vi "itc Hg box controller.vi"(6 "Log File Path":path, 7 "itc box action":T2=enum."read sweep table", 8 "error in":errorcluster, 9 "Sweep Table In":dbl[][](array[numeric])=[[650.0, 1334.0, 30.0], [300.0, 1334.0, 0.0], [0.0, 0.0, 0.0], [0.0, 0.0, 0.0], [0.0, 0.0, 0.0], [0.0, 0.0, 0.0], [0.0, 0.0, 0.0], [0.0, 0.0, 0.0], [0.0, 0.0, 0.0], [0.0, 0.0, 0.0], [0.0, 0.0, 0.0], [300.0, 0.0, 0.0], [0.0, 0.0, 0.0], [0.0, 0.0, 0.0], [0.0, 0.0, 0.0], [300.0, 0.0, 0.0]], 10 "input":dbl=300.0, 11 "VISA resource name":refnum<visa-resource-name>="GPIB0::23::INSTR") -> (0 "error out":errorcluster, 1 "Sweep Table":dbl[][](array[numeric])=[[650.0, 1334.0, 30.0], [300.0, 1334.0, 0.0], [0.0, 0.0, 0.0], [0.0, 0.0, 0.0], [0.0, 0.0, 0.0], [0.0, 0.0, 0.0], [0.0, 0.0, 0.0], [0.0, 0.0, 0.0], [0.0, 0.0, 0.0], [0.0, 0.0, 0.0], [0.0, 0.0, 0.0], [300.0, 0.0, 0.0], [0.0, 0.0, 0.0], [0.0, 0.0, 0.0], [0.0, 0.0, 0.0], [300.0, 0.0, 0.0]], 2 "itc box state OUT":T1={"ITC503 Address"="GPIB0::15::INSTR", "ITC temperature"=0.0, "ITC set temperature"=300.0, "heater"=300.0, "gas flow"=1.6, "P"=0.0, "D"=10.0, "I"=0.1, "ITC state"="X0A1C2S01H1L0\r", "nonzero temperature"=0.0, "Magn Field (T)"=0.0})   [LabVIEW 2015]
uses:
  itc 503 box - control.ctl
  itc 503 box state.ctl
  Q - not nan -- real.vi
panel:
  out "F-format string":string
  out "enabled state":enum16{"disabled", "enabled"}(ring)
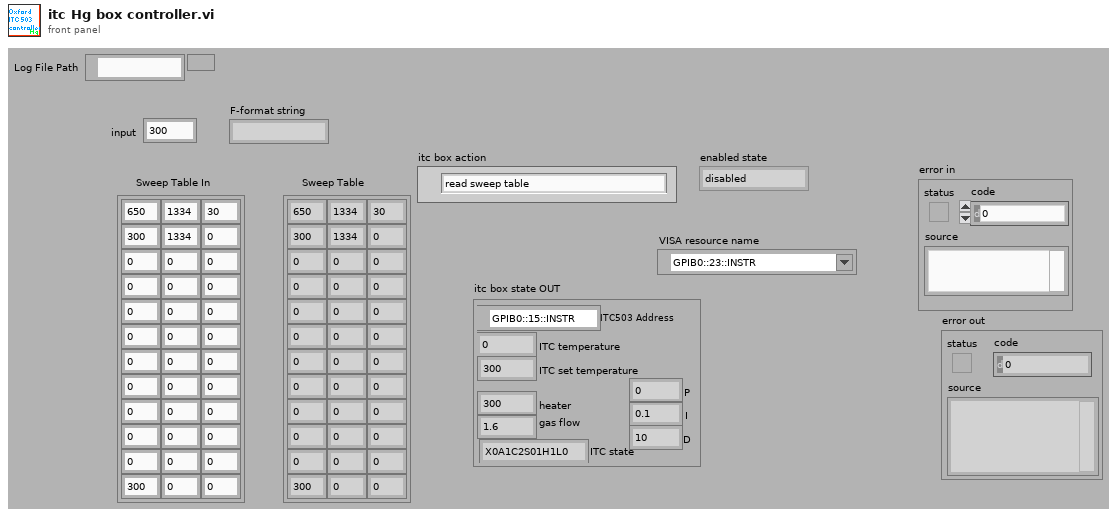
[diagram p1: front panel]
types:
  T1 = typedef "itc 503 box state.ctl" = cluster{"ITC503 Address":refnum<visa-resource-name>, "ITC temperature":dbl, "ITC set temperature":dbl, "heater":dbl, "gas flow":dbl, "P":dbl, "D":dbl, "I":dbl, "ITC state":string, "nonzero temperature":dbl, "Magn Field (T)":dbl}
  T2 = typedef "itc 503 box - control.ctl" = enum16{"heater manual and zero", "heater auto", "upload D", "upload I", "upload P", "shut off", "init", "read sweep table", "disable", "enable", "read state", "set gas to", "stop sweep", "start sweep", "test", "set temperature to", "write sweep table", "-void", "set heater to"}
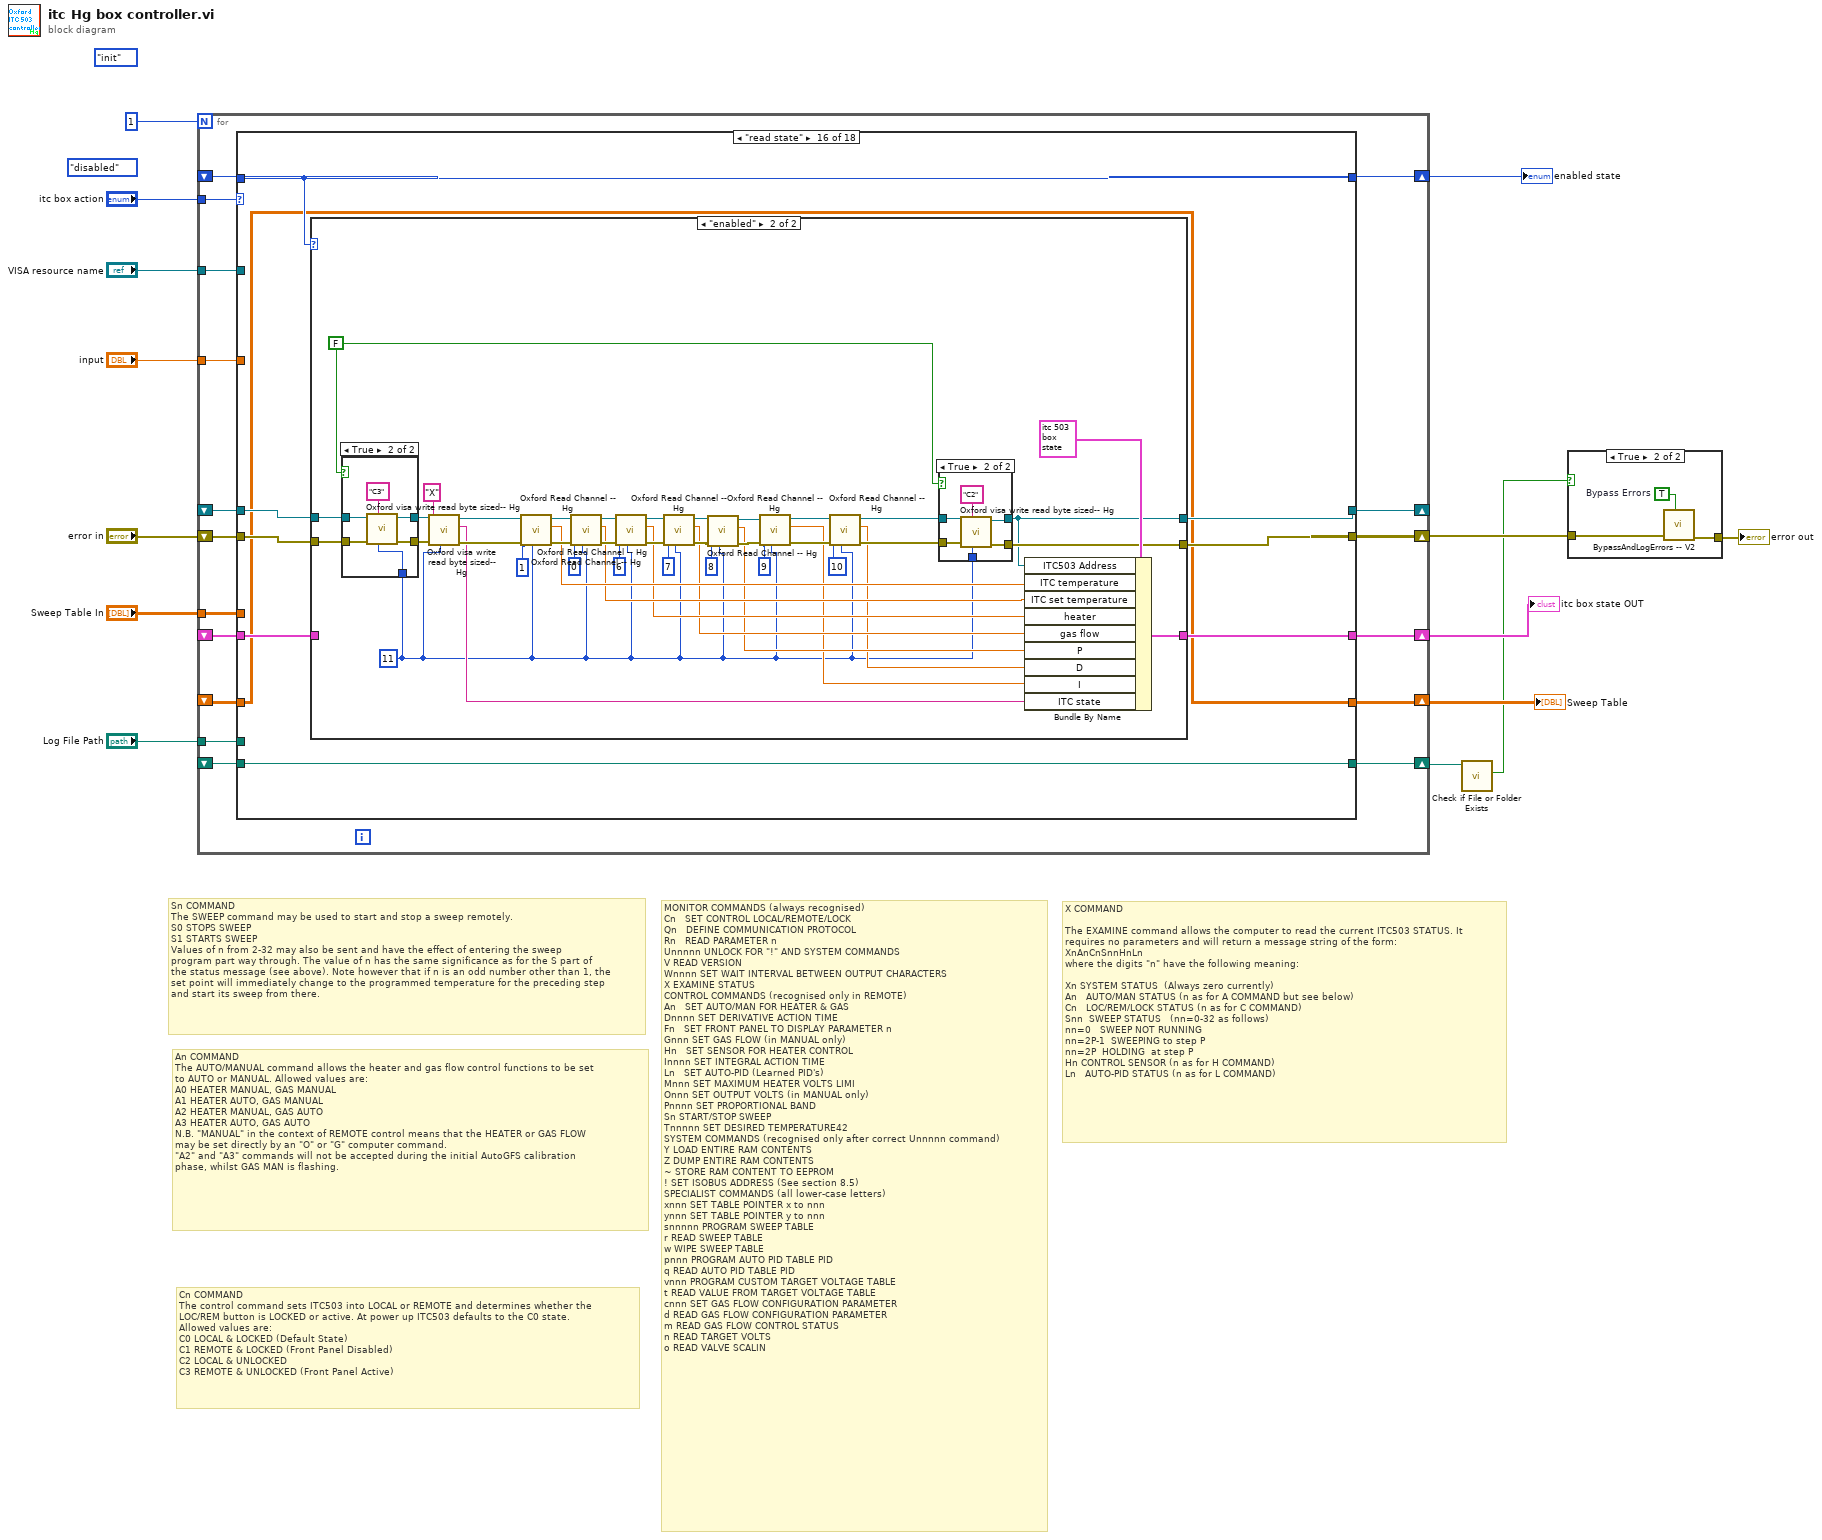
[diagram p0: block diagram]
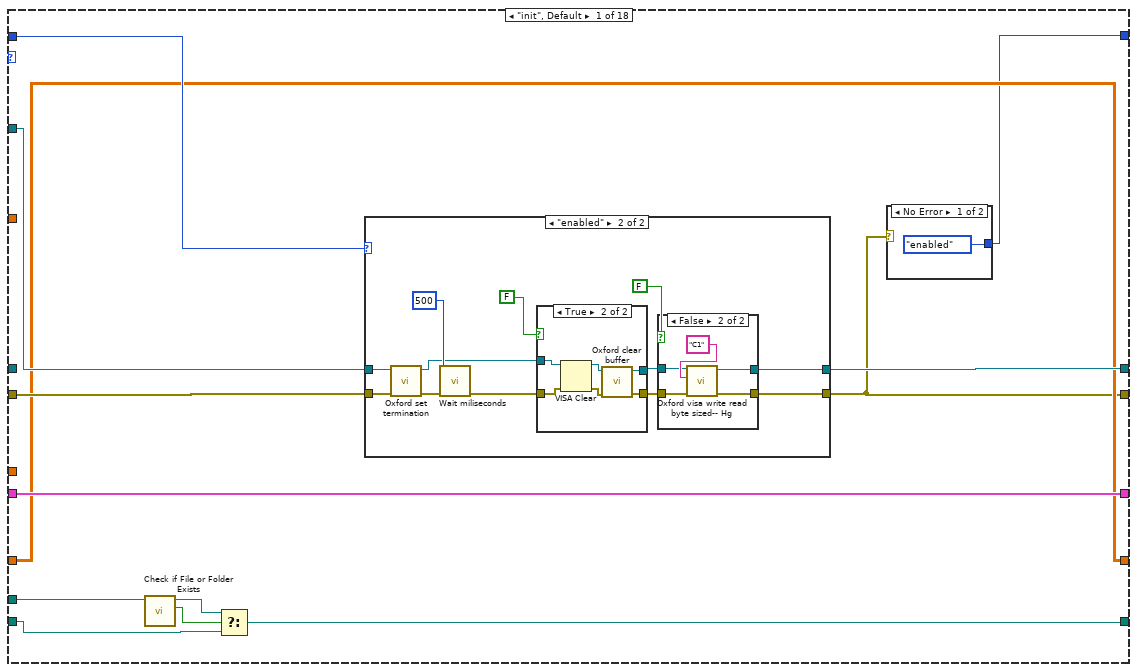
[diagram p3: hidden frame]
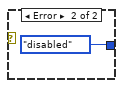
[diagram p4: hidden frame]
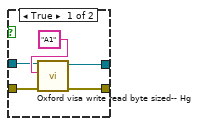
[diagram p7: hidden frame]
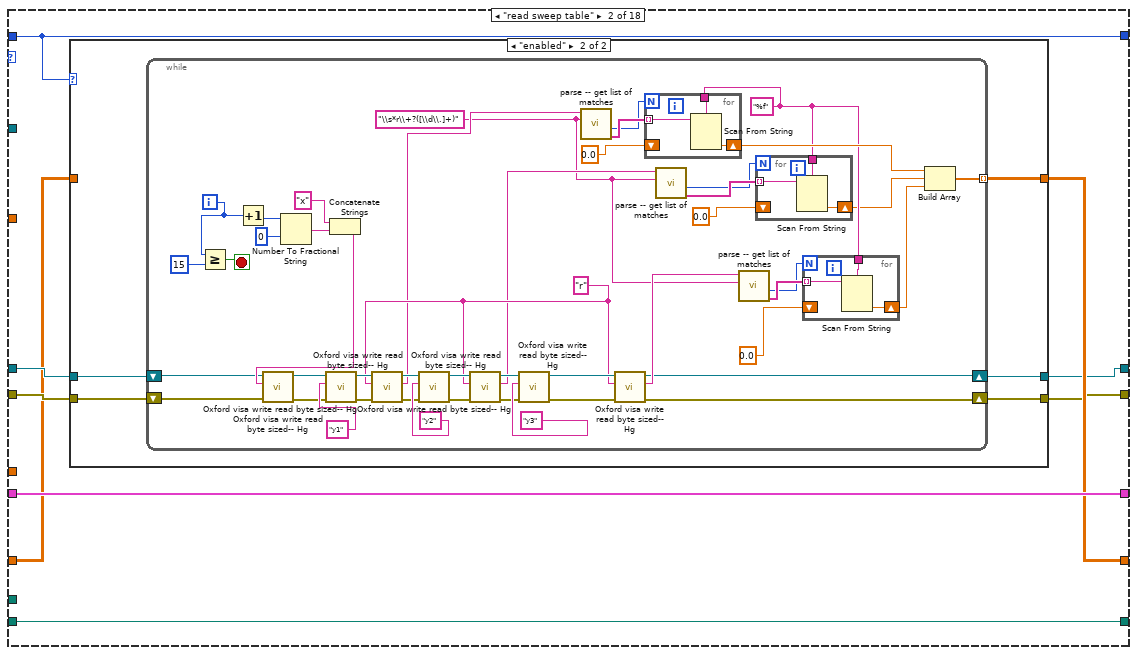
[diagram p8: hidden frame]
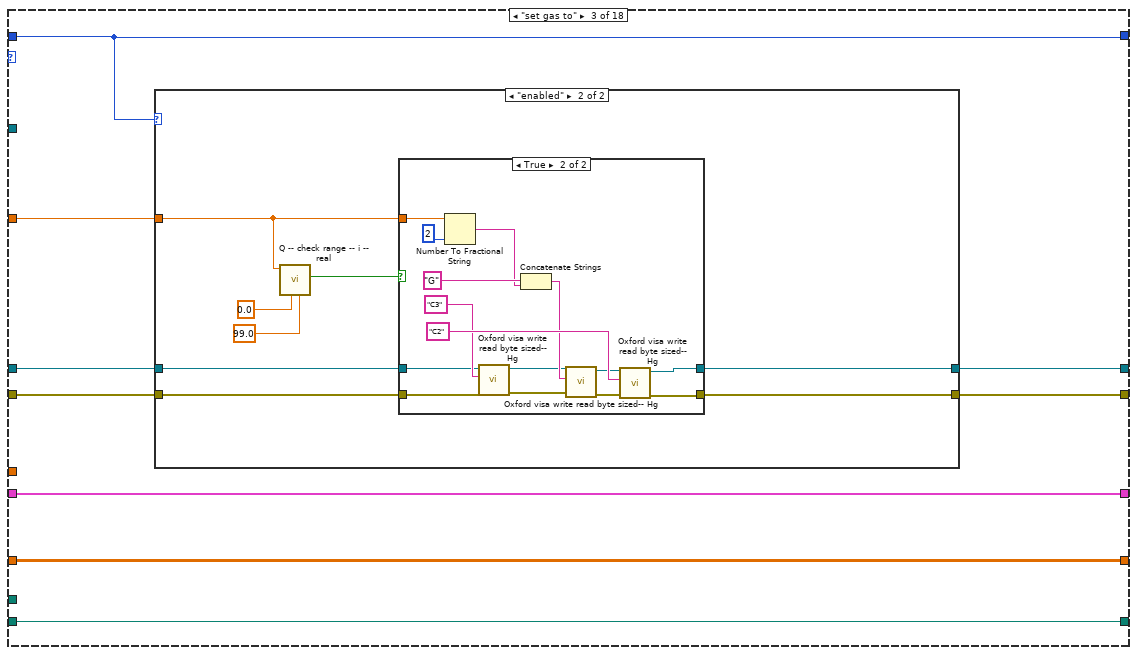
[diagram p10: hidden frame]
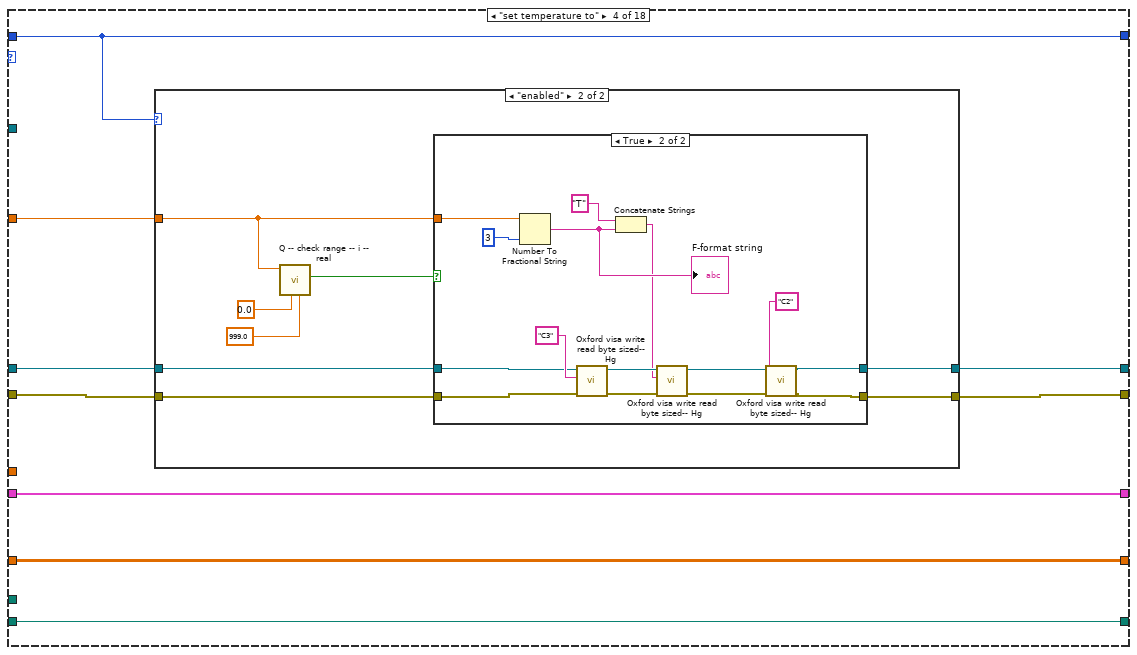
[diagram p13: hidden frame]
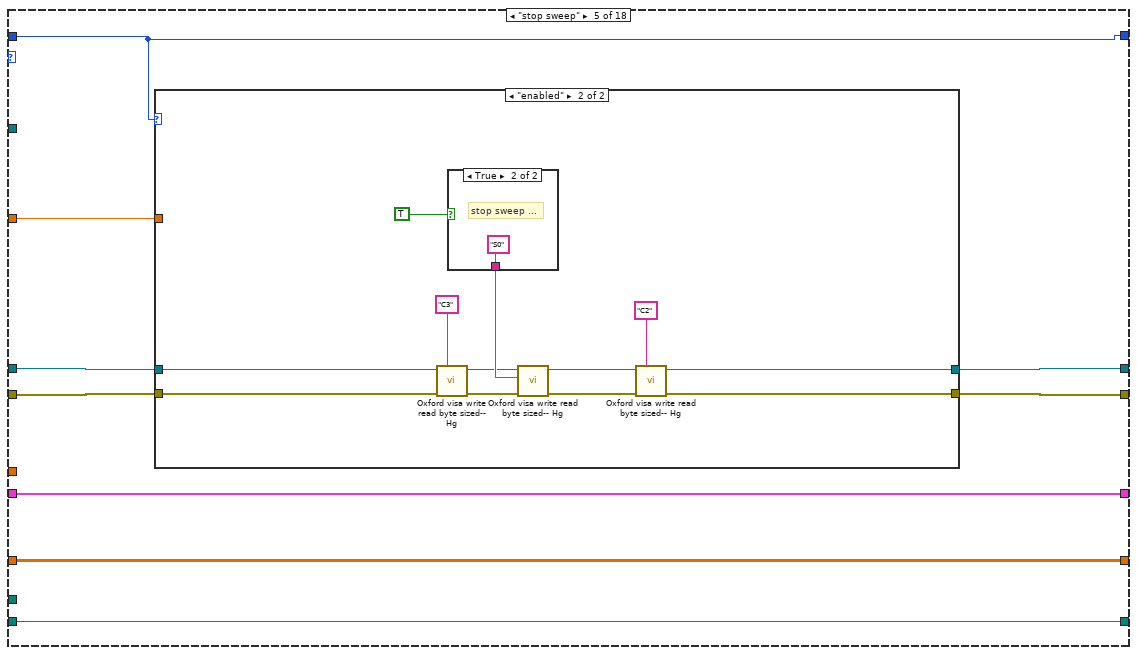
[diagram p16: hidden frame]
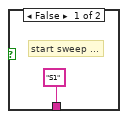
[diagram p18: hidden frame]
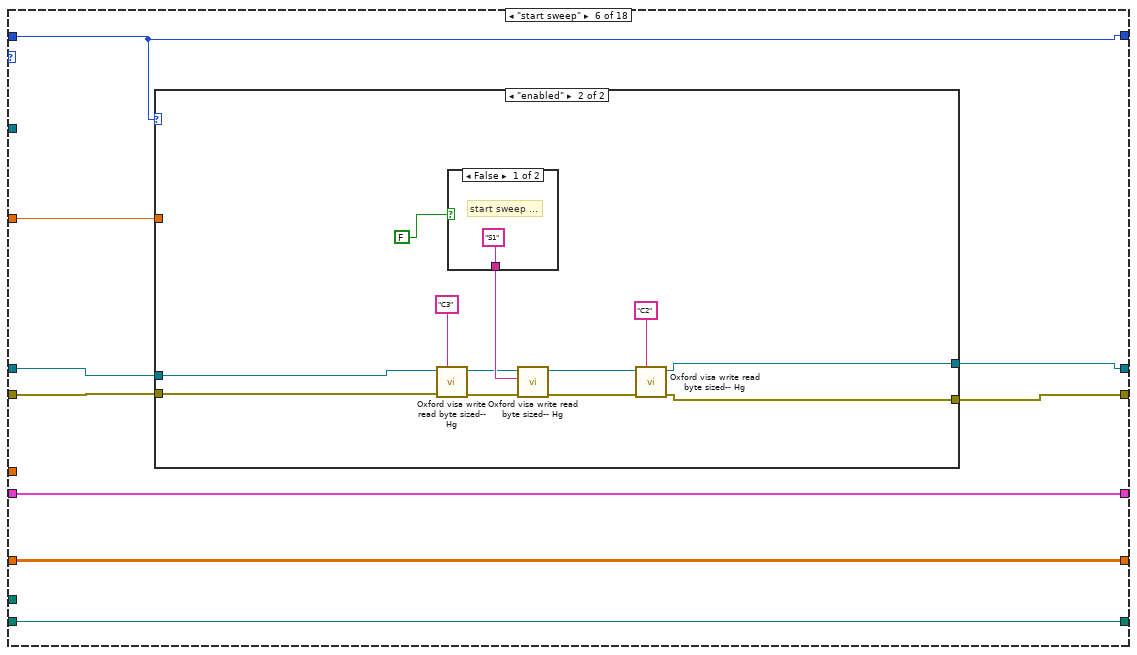
[diagram p19: hidden frame]
diagram:
  (unwired) enum16{"disabled", "enabled"}."disabled" ("disable interaction with itc  2")
  (unwired) itc_503_box_-_control."init" ("itc box action")
  # "Cn COMMAND\nThe control command sets ITC503 into LOCAL or REMOTE and determines whether the\nLOC/REM button is LOCKED or active. At power up ITC503 defaults to the C0 state.\nAllowed values are:\nC0 LOCAL & LOCKED (Default State)\nC1 REMOTE & LOCKED (Front Panel Disabled)\nC2 LOCAL & UNLOCKED\nC3 REMOTE & UNLOCKED (Front Panel Active)"
  # "An COMMAND\nThe AUTO/MANUAL command allows the heater and gas flow control functions to be set\nto AUTO or MANUAL. Allowed values are:\nA0 HEATER MANUAL, GAS MANUAL\nA1 HEATER AUTO, GAS MANUAL\nA2 HEATER MANUAL, GAS AUTO\nA3 HEATER AUTO, GAS AUTO\nN.B. \"MANUAL\" in the context of REMOTE control means that the HEATER or GAS FLOW\nmay be set directly by an \"O\" or \"G\" computer command.\n\"A2\" and \"A3\" commands will not be accepted during the initial AutoGFS calibration\nphase, whilst GAS MAN is flashing."
  # "MONITOR COMMANDS (always recognised)\nCn   SET CONTROL LOCAL/REMOTE/LOCK\nQn   DEFINE COMMUNICATION PROTOCOL\nRn   READ PARAMETER n\nUnnnnn UNLOCK FOR \"!\" AND SYSTEM COMMANDS\nV READ VERSION\nWnnnn SET WAIT INTERVAL BETWEEN OUTPUT CHARACTERS\nX EXAMINE STATUS\nCONTROL COMMANDS (recognised only in REMOTE)\nAn   SET AUTO/MAN FOR HEATER & GAS\nDnnnn SET DERIVATIVE ACTION TIME\nFn   SET FRONT PANEL TO DISPLAY PARAMETER n\nGnnn SET GAS FLOW (in MANUAL only)\nHn   SET SENSOR FOR HEATER CONTROL\nInnnn SET INTEGRAL ACTION TIME\nLn   SET AUTO-PID (Learned PID's)\nMnnn SET MAXIMUM HEATER VOLTS LIMI\nOnnn SET OUTPUT VOLTS (in MANUAL only)\nPnnnn SET PROPORTIONAL BAND\nSn START/STOP SWEEP\nTnnnnn SET DESIRED TEMPERATURE42\nSYSTEM COMMANDS (recognised only after correct Unnnnn command)\nY LOAD ENTIRE RAM CONTENTS\nZ DUMP ENTIRE RAM CONTENTS\n~ STORE RAM CONTENT TO EEPROM\n! SET ISOBUS ADDRESS (See section 8.5)\nSPECIALIST COMMANDS (all lower-case letters)\nxnnn SET TABLE POINTER x to nnn\nynnn SET TABLE POINTER y to nnn\nsnnnnn PROGRAM SWEEP TABLE\nr READ SWEEP TABLE\nw WIPE SWEEP TABLE\npnnn PROGRAM AUTO PID TABLE PID\nq READ AUTO PID TABLE PID\nvnnn PROGRAM CUSTOM TARGET VOLTAGE TABLE\nt READ VALUE FROM TARGET VOLTAGE TABLE\ncnnn SET GAS FLOW CONFIGURATION PARAMETER\nd READ GAS FLOW CONFIGURATION PARAMETER\nm READ GAS FLOW CONTROL STATUS\nn READ TARGET VOLTS\no READ VALVE SCALIN"
  # "X COMMAND\n\nThe EXAMINE command allows the computer to read the current ITC503 STATUS. It\nrequires no parameters and will return a message string of the form:\nXnAnCnSnnHnLn\nwhere the digits \"n\" have the following meaning:\n\nXn SYSTEM STATUS  (Always zero currently)\nAn   AUTO/MAN STATUS (n as for A COMMAND but see below)\nCn   LOC/REM/LOCK STATUS (n as for C COMMAND)\nSnn  SWEEP STATUS   (nn=0-32 as follows)\nnn=0   SWEEP NOT RUNNING\nnn=2P-1  SWEEPING to step P\nnn=2P  HOLDING  at step P\nHn CONTROL SENSOR (n as for H COMMAND)\nLn   AUTO-PID STATUS (n as for L COMMAND)"
  # "Sn COMMAND\nThe SWEEP command may be used to start and stop a sweep remotely.\nS0 STOPS SWEEP\nS1 STARTS SWEEP\nValues of n from 2-32 may also be sent and have the effect of entering the sweep\nprogram part way through. The value of n has the same significance as for the S part of\nthe status message (see above). Note however that if n is an odd number other than 1, the\nset point will immediately change to the programmed temperature for the preceding step\nand start its sweep from there."
  n1 = for {
    N: 1 -> [_]
    tunnel: "itc box action" -> [w31]
    shift-right: [w29] -> _
    shift-left: _ -> [w30]
    tunnel: "VISA resource name" -> [w28]
    shift-right: [w27] -> w7
    shift-left: _ -> [w26]
    shift-right: [w25] -> w6
    shift-left: _ -> [w23]
    shift-right: [w18] -> w4
    shift-left: "error in" -> [w24]
    shift-right: [w22] -> w10
    shift-left: _ -> [w21]
    tunnel: "input" -> [w20]
    tunnel: "Sweep Table In" -> [w19]
    tunnel: "Log File Path" -> [w17]
    shift-right: [w16] -> w2
    shift-left: _ -> [w15]
    n2 = case shown="\"read state\"" w31 {
      tunnel: w30 -> [_ w85 w158 w194 w230 w255 w280 w306 w332 w358 w380 w405 w434 w478 w490 w507 w574 w580]
      tunnel: [w44 w82 w155 w191 w227 w252 w277 w303 w329 w355 w377 w402 w431 w478 w487 w504 w574 w580] -> w29
      tunnel: w28 -> [w43 _ _ _ _ _ _ _ _ _ _ _ _ _ _ _ _ _]
      tunnel: [w37 w81 w152 w188 w224 w249 w274 w300 w326 w352 w374 w399 w428 w479 w484 w503 enum16{"disabled", "enabled"}."disabled" ("disable interaction with itc  2") enum16{"disabled", "enabled"}."enabled" ("disable interaction with itc  2")] -> w27
      tunnel: w26 -> [w42 w81 w152 w188 w224 w249 w274 w300 w326 w352 w374 w399 w428 w479 w484 w503 _ _]
      tunnel: [w40 w87 w154 w190 w226 w251 w276 w302 w328 w354 w376 w401 w430 w481 w486 w508 w572 w578] -> w25
      tunnel: w24 -> [w41 w84 w157 w193 w229 w254 w279 w305 w331 w357 w379 w404 w433 w477 w489 w506 w573 w579]
      tunnel: [w38 w83 w156 w192 w228 w253 w278 w304 w330 w356 w378 w403 w432 w477 w488 w505 w573 w579] -> w18
      tunnel: w23 -> [w40 w87 w154 w190 w226 w251 w276 w302 w328 w354 w376 w401 w430 w481 w486 w502 w572 w578]
      tunnel: [w39 w86 w153 w189 w225 w250 w275 w301 w327 w353 w375 w400 w429 w480 w485 w501 w571 w577] -> w22
      tunnel: w21 -> [w39 w80 w153 w189 w225 w250 w275 w301 w327 w353 w375 w400 w429 w480 w485 w501 w571 w577]
      tunnel: w20 -> [_ _ w159 w195 w231 w256 w281 w307 w333 w359 w381 w406 w435 _ w491 _ _ _]
      tunnel: w19 -> [_ _ _ _ _ _ _ _ _ _ _ _ _ _ w483 _ _ _]
      tunnel: w17 -> [w36 _ _ _ _ _ _ _ _ _ _ _ _ _ _ _ _ _]
      tunnel: [w33 w79 w151 w187 w223 w248 w273 w299 w325 w351 w373 w398 w427 w476 w482 w500 w570 w576] -> w16
      tunnel: w15 -> [w32 w79 w151 w187 w223 w248 w273 w299 w325 w351 w373 w398 w427 w476 w482 w500 w570 w576]
      frame "init", Default {
        n3 = call <vilib>:"Check if File or Folder Exists.vi"("path"=w36) -> ("file or folder exists?"=w35:bool, "dup path"=w34:path)  [unwired: 8 in, 1 out]
        n4 = Select(t=w34, s=w35, f=w32) -> (s? t:f=w33:path)
        n5 = case shown="\"enabled\"" w42 {
          tunnel: [w48 w57] -> w44
          tunnel: w43 -> [w48 w54]
          tunnel: w41 -> [w47 w53]
          tunnel: [w47 w56] -> w38
          frame "disabled", Default {
          }
          frame "enabled" {
            n6 = call "Oxford set termination.vi"("error in (no error)"=w53, "VISA resource name"=w54) -> ("error out"=w50:errorcluster, "VISA resource name out"=w49:refnum<visa-resource-name>)  [unwired: 8 in]
            n7 = call "Wait miliseconds.vi"("error in (no error)"=w50, "milliseconds to wait"=u32 500) -> ("error out"=w52:errorcluster)  [unwired: 8 in, 1 out]
            n8 = case shown="True" FALSE {
              tunnel: [w61 w68] -> w60
              tunnel: [w62 w67] -> w59
              tunnel: w52 -> [w61 w63]
              tunnel: w49 -> [w62 w66]
              frame False {
              }
              frame True {
                n9 = VISA Clear(VISA resource name=w66, error in (no error)=w63) -> (VISA resource name out=w65:refnum<visa-resource-name>, error out=w64:errorcluster)
                n10 = call "Oxford clear buffer.vi"("error in (no error)"=w64, "VISA resource name"=w65) -> ("error out"=w68:errorcluster, "VISA resource name out"=w67:refnum<visa-resource-name>)  [unwired: 6 in, 2 out]
              }
            }
            n11 = case shown="False" FALSE {
              tunnel: w60 -> [w72 w77]
              tunnel: w59 -> [w71 w76]
              tunnel: [w70 w75] -> w57
              tunnel: [w69 w74] -> w56
              frame True {
                n12 = call "Oxford visa write read byte sized-- Hg.vi"("error in (no error)"=w72, "write buffer"="A1" ("Command"), "VISA resource name"=w71) -> ("error out"=w69:errorcluster, "VISA resource name out"=w70:refnum<visa-resource-name>)  [unwired: 6 in, 1 out]
              }
              frame False {
                n13 = call "Oxford visa write read byte sized-- Hg.vi"("error in (no error)"=w77, "write buffer"="C1" ("Command"), "VISA resource name"=w76) -> ("error out"=w74:errorcluster, "VISA resource name out"=w75:refnum<visa-resource-name>)  [unwired: 6 in, 1 out]
              }
            }
          }
        }
        n14 = case shown="No Error" w38 {
          tunnel: [enum16{"disabled", "enabled"}."enabled" ("disable interaction with itc  2") enum16{"disabled", "enabled"}."disabled" ("disable interaction with itc  2")] -> w37
          frame No Error {
          }
          frame Error {
          }
        }
      }
      frame "read sweep table" {
        n15 = case shown="\"enabled\"" w81 {
          tunnel: [w88 w95] -> w86
          tunnel: w85 -> [w90 w94]
          tunnel: w84 -> [w89 w93]
          tunnel: [w89 w92] -> w83
          tunnel: [w90 w91] -> w82
          tunnel: w80 -> [w88 _]
          frame "disabled", Default {
          }
          frame "enabled" {
            n16 = while {
              tunnel: [w117] -> w95 mode=indexing
              shift-right: [w97] -> w91
              shift-left: w94 -> [w120]
              shift-right: [w96] -> w92
              shift-left: w93 -> [w127]
              i -> [w115]
              stop <- w114 stop-if-true
              w101 = "\\s*r\\+?([\\d\\.]+)" ("format string")
              w100 = "%f" ("format string")
              w119 = "r" ("string")
              n17 = Greater Or Equal?(x=w115, y=15) -> (x >= y?=w114:bool)
              n18 = Increment(x=w115) -> (x+1=w141:i32)
              n19 = Number To Fractional String(number=w141, precision (6)=i16 0) -> (F-format string=w138:string)  [unwired: 2 in]
              n20 = Concatenate Strings("x" ("string"), w138) -> (w137:string)
              n21 = call "Oxford visa write read byte sized-- Hg.vi"("error in (no error)"=w127, "write buffer"=w137, "VISA resource name"=w120) -> ("error out"=w133:errorcluster, "VISA resource name out"=w121:refnum<visa-resource-name>)  [unwired: 6 in, 1 out]
              n22 = call "Oxford visa write read byte sized-- Hg.vi"("error in (no error)"=w133, "write buffer"="y1" ("string"), "VISA resource name"=w121) -> ("error out"=w132:errorcluster, "VISA resource name out"=w122:refnum<visa-resource-name>)  [unwired: 6 in, 1 out]
              n23 = call "Oxford visa write read byte sized-- Hg.vi"("error in (no error)"=w132, "write buffer"=w119, "VISA resource name"=w122) -> ("error out"=w131:errorcluster, "read buffer"=w113:string, "VISA resource name out"=w123:refnum<visa-resource-name>)  [unwired: 6 in]
              n24 = call "Oxford visa write read byte sized-- Hg.vi"("error in (no error)"=w131, "write buffer"="y2" ("string"), "VISA resource name"=w123) -> ("error out"=w130:errorcluster, "VISA resource name out"=w126:refnum<visa-resource-name>)  [unwired: 6 in, 1 out]
              n25 = call "Oxford visa write read byte sized-- Hg.vi"("error in (no error)"=w130, "write buffer"=w119, "VISA resource name"=w126) -> ("error out"=w129:errorcluster, "read buffer"=w102:string, "VISA resource name out"=w125:refnum<visa-resource-name>)  [unwired: 6 in]
              n26 = call "Oxford visa write read byte sized-- Hg.vi"("error in (no error)"=w129, "write buffer"="y3" ("string"), "VISA resource name"=w125) -> ("error out"=w128:errorcluster, "VISA resource name out"=w124:refnum<visa-resource-name>)  [unwired: 6 in, 1 out]
              n27 = call "parse -- get list of matches.vi"("regexp"=w101, "string"=w113) -> ("Array"=w112:string[], "number of free elastic constants"=w111:i32)  [unwired: 7 in, 1 out]
              n28 = call "Oxford visa write read byte sized-- Hg.vi"("error in (no error)"=w128, "write buffer"=w119, "VISA resource name"=w124) -> ("error out"=w96:errorcluster, "read buffer"=w103:string, "VISA resource name out"=w97:refnum<visa-resource-name>)  [unwired: 6 in]
              n29 = for {
                N: w111 -> [_]
                tunnel: w100 -> [w149]
                tunnel: w112 -> [w148] mode=indexing
                shift-right: [w150] -> w118
                shift-left: 0.0 -> [_]
                n30 = Scan From String(format string=w149, input string=w148) -> (output 1=w150:dbl)  [unwired: 3 in, 3 out]
              }
              n31 = call "parse -- get list of matches.vi"("regexp"=w101, "string"=w102) -> ("Array"=w109:string[], "number of free elastic constants"=w108:i32)  [unwired: 7 in, 1 out]
              n32 = call "parse -- get list of matches.vi"("regexp"=w101, "string"=w103) -> ("Array"=w106:string[], "number of free elastic constants"=w105:i32)  [unwired: 7 in, 1 out]
              n33 = for {
                N: w108 -> [_]
                tunnel: w109 -> [w146] mode=indexing
                shift-right: [w147] -> w98
                shift-left: 0.0 -> [_]
                tunnel: w100 -> [w145]
                n34 = Scan From String(format string=w145, input string=w146) -> (output 1=w147:dbl)  [unwired: 3 in, 3 out]
              }
              n35 = for {
                N: w105 -> [_]
                tunnel: w106 -> [w143] mode=indexing
                shift-right: [w144] -> w99
                shift-left: 0.0 -> [_]
                tunnel: w100 -> [w142]
                n36 = Scan From String(format string=w142, input string=w143) -> (output 1=w144:dbl)  [unwired: 3 in, 3 out]
              }
              n37 = Build Array(w118, w98, w99) -> (w117:dbl[])
            }
          }
        }
      }
      frame "set gas to" {
        n38 = case shown="\"enabled\"" w152 {
          tunnel: w159 -> [_ w167]
          tunnel: w158 -> [w161 w165]
          tunnel: w157 -> [w160 w164]
          tunnel: [w160 w163] -> w156
          tunnel: [w161 w162] -> w155
          frame "disabled", Default {
          }
          frame "enabled" {
            n39 = call "Q -- check range -- i -- real.vi"("upper"=99.0, "lower"=0.0, "number"=w167) -> ("in range?"=w166:bool)  [unwired: 6 in, 2 out]
            n40 = case shown="True" w166 {
              tunnel: w164 -> [w171 w178]
              tunnel: [w171 w177] -> w163
              tunnel: [w170 w174] -> w162
              tunnel: w167 -> [_ w173]
              tunnel: w165 -> [w170 w172]
              frame False {
                # "need to rize some kind of error ..."
              }
              frame True {
                n41 = Number To Fractional String(number=w173, precision (6)=i16 2) -> (F-format string=w183:string)  [unwired: 2 in]
                n42 = call "Oxford visa write read byte sized-- Hg.vi"("error in (no error)"=w178, "write buffer"="C3" ("Command"), "VISA resource name"=w172) -> ("error out"=w182:errorcluster, "VISA resource name out"=w176:refnum<visa-resource-name>)  [unwired: 6 in, 1 out]
                n43 = Concatenate Strings("G" ("string"), w183) -> (w180:string)
                n44 = call "Oxford visa write read byte sized-- Hg.vi"("error in (no error)"=w182, "write buffer"=w180, "VISA resource name"=w176) -> ("error out"=w181:errorcluster, "VISA resource name out"=w175:refnum<visa-resource-name>)  [unwired: 6 in, 1 out]
                n45 = call "Oxford visa write read byte sized-- Hg.vi"("error in (no error)"=w181, "write buffer"="C2" ("Command"), "VISA resource name"=w175) -> ("error out"=w177:errorcluster, "VISA resource name out"=w174:refnum<visa-resource-name>)  [unwired: 6 in, 1 out]
              }
            }
          }
        }
      }
      frame "set temperature to" {
        n46 = case shown="\"enabled\"" w188 {
          tunnel: w195 -> [_ w199]
          tunnel: w194 -> [w197 w203]
          tunnel: w193 -> [w196 w198]
          tunnel: [w196 w201] -> w192
          tunnel: [w197 w202] -> w191
          frame "disabled", Default {
          }
          frame "enabled" {
            n47 = call "Q -- check range -- i -- real.vi"("upper"=999.0, "lower"=0.0, "number"=w199) -> ("in range?"=w200:bool)  [unwired: 6 in, 2 out]
            n48 = case shown="True" w200 {
              tunnel: w203 -> [w207 w212]
              tunnel: [w207 w211] -> w202
              tunnel: [w206 w210] -> w201
              tunnel: w199 -> [_ w209]
              tunnel: w198 -> [w206 w208]
              frame False {
              }
              frame True {
                n49 = Number To Fractional String(number=w209, precision (6)=i16 3) -> (F-format string=w217:string)  [unwired: 2 in]
                "F-format string" <- w217
                n50 = call "Oxford visa write read byte sized-- Hg.vi"("error in (no error)"=w208, "write buffer"="C3" ("Command"), "VISA resource name"=w212) -> ("error out"=w222:errorcluster, "VISA resource name out"=w221:refnum<visa-resource-name>)  [unwired: 6 in, 1 out]
                n51 = Concatenate Strings("T" ("Command"), w217) -> (w215:string)
                n52 = call "Oxford visa write read byte sized-- Hg.vi"("error in (no error)"=w222, "write buffer"=w215, "VISA resource name"=w221) -> ("error out"=w213:errorcluster, "VISA resource name out"=w214:refnum<visa-resource-name>)  [unwired: 6 in, 1 out]
                n53 = call "Oxford visa write read byte sized-- Hg.vi"("error in (no error)"=w213, "write buffer"="C2" ("Command"), "VISA resource name"=w214) -> ("error out"=w210:errorcluster, "VISA resource name out"=w211:refnum<visa-resource-name>)  [unwired: 6 in, 1 out]
              }
            }
          }
        }
      }
      frame "stop sweep" {
        n54 = case shown="\"enabled\"" w224 {
          tunnel: w231 -> [_ _]
          tunnel: w230 -> [w233 w234]
          tunnel: w229 -> [w232 w237]
          tunnel: [w232 w236] -> w228
          tunnel: [w233 w235] -> w227
          frame "disabled", Default {
          }
          frame "enabled" {
            n55 = call "Oxford visa write read byte sized-- Hg.vi"("error in (no error)"=w237, "write buffer"="C3" ("Command"), "VISA resource name"=w234) -> ("error out"=w241:errorcluster, "VISA resource name out"=w240:refnum<visa-resource-name>)  [unwired: 6 in, 1 out]
            n56 = case shown="True" TRUE {
              tunnel: ["S1" ("write buffer") "S0" ("write buffer")] -> w245
              frame False {
                # "start sweep ..."
              }
              frame True {
                # "stop sweep ..."
              }
            }
            n57 = call "Oxford visa write read byte sized-- Hg.vi"("error in (no error)"=w241, "write buffer"=w245, "VISA resource name"=w240) -> ("error out"=w244:errorcluster, "VISA resource name out"=w242:refnum<visa-resource-name>)  [unwired: 6 in, 1 out]
            n58 = call "Oxford visa write read byte sized-- Hg.vi"("error in (no error)"=w244, "write buffer"="C2" ("Command"), "VISA resource name"=w242) -> ("error out"=w236:errorcluster, "VISA resource name out"=w235:refnum<visa-resource-name>)  [unwired: 6 in, 1 out]
          }
        }
      }
      frame "start sweep" {
        n59 = case shown="\"enabled\"" w249 {
          tunnel: w256 -> [_ _]
          tunnel: w255 -> [w258 w259]
          tunnel: w254 -> [w257 w262]
          tunnel: [w257 w261] -> w253
          tunnel: [w258 w260] -> w252
          frame "disabled", Default {
          }
          frame "enabled" {
            n60 = call "Oxford visa write read byte sized-- Hg.vi"("error in (no error)"=w262, "write buffer"="C3" ("Command"), "VISA resource name"=w259) -> ("error out"=w266:errorcluster, "VISA resource name out"=w265:refnum<visa-resource-name>)  [unwired: 6 in, 1 out]
            n61 = case shown="False" FALSE {
              tunnel: ["S1" ("write buffer") "S0" ("write buffer")] -> w270
              frame False {
                # "start sweep ..."
              }
              frame True {
                # "stop sweep ..."
              }
            }
            n62 = call "Oxford visa write read byte sized-- Hg.vi"("error in (no error)"=w266, "write buffer"=w270, "VISA resource name"=w265) -> ("error out"=w269:errorcluster, "VISA resource name out"=w267:refnum<visa-resource-name>)  [unwired: 6 in, 1 out]
            n63 = call "Oxford visa write read byte sized-- Hg.vi"("error in (no error)"=w269, "write buffer"="C2" ("Command"), "VISA resource name"=w267) -> ("error out"=w261:errorcluster, "VISA resource name out"=w260:refnum<visa-resource-name>)  [unwired: 6 in, 1 out]
          }
        }
      }
      frame "upload P" {
        n64 = case shown="\"enabled\"" w274 {
          tunnel: w281 -> [_ w284]
          tunnel: w280 -> [w283 w286]
          tunnel: w279 -> [w282 w287]
          tunnel: [w282 w289] -> w278
          tunnel: [w283 w290] -> w277
          frame "disabled", Default {
          }
          frame "enabled" {
            n65 = Number To Fractional String(number=w284, precision (6)=i16 4 ("width (-)")) -> (F-format string=w296:string)  [unwired: 2 in]
            n66 = call "Oxford visa write read byte sized-- Hg.vi"("error in (no error)"=w287, "write buffer"="C3" ("Command"), "VISA resource name"=w286) -> ("error out"=w295:errorcluster, "VISA resource name out"=w292:refnum<visa-resource-name>)  [unwired: 6 in, 1 out]
            n67 = Concatenate Strings("P" ("string"), w296) -> (w298:string)
            n68 = call "Oxford visa write read byte sized-- Hg.vi"("error in (no error)"=w295, "write buffer"=w298, "VISA resource name"=w292) -> ("error out"=w288:errorcluster, "VISA resource name out"=w291:refnum<visa-resource-name>)  [unwired: 6 in, 1 out]
            n69 = call "Oxford visa write read byte sized-- Hg.vi"("error in (no error)"=w288, "write buffer"="C2" ("Command"), "VISA resource name"=w291) -> ("error out"=w289:errorcluster, "VISA resource name out"=w290:refnum<visa-resource-name>)  [unwired: 6 in, 1 out]
          }
        }
      }
      frame "upload I" {
        n70 = case shown="\"enabled\"" w300 {
          tunnel: w307 -> [_ w310]
          tunnel: w306 -> [w309 w312]
          tunnel: w305 -> [w308 w313]
          tunnel: [w308 w315] -> w304
          tunnel: [w309 w316] -> w303
          frame "disabled", Default {
          }
          frame "enabled" {
            n71 = Number To Fractional String(number=w310, precision (6)=i16 4 ("width (-)")) -> (F-format string=w322:string)  [unwired: 2 in]
            n72 = call "Oxford visa write read byte sized-- Hg.vi"("error in (no error)"=w313, "write buffer"="C3" ("Command"), "VISA resource name"=w312) -> ("error out"=w321:errorcluster, "VISA resource name out"=w318:refnum<visa-resource-name>)  [unwired: 6 in, 1 out]
            n73 = Concatenate Strings("I" ("string"), w322) -> (w324:string)
            n74 = call "Oxford visa write read byte sized-- Hg.vi"("error in (no error)"=w321, "write buffer"=w324, "VISA resource name"=w318) -> ("error out"=w314:errorcluster, "VISA resource name out"=w317:refnum<visa-resource-name>)  [unwired: 6 in, 1 out]
            n75 = call "Oxford visa write read byte sized-- Hg.vi"("error in (no error)"=w314, "write buffer"="C2" ("Command"), "VISA resource name"=w317) -> ("error out"=w315:errorcluster, "VISA resource name out"=w316:refnum<visa-resource-name>)  [unwired: 6 in, 1 out]
          }
        }
      }
      frame "upload D" {
        n76 = case shown="\"enabled\"" w326 {
          tunnel: w333 -> [_ w336]
          tunnel: w332 -> [w335 w338]
          tunnel: w331 -> [w334 w339]
          tunnel: [w334 w341] -> w330
          tunnel: [w335 w342] -> w329
          frame "disabled", Default {
          }
          frame "enabled" {
            n77 = Number To Fractional String(number=w336, precision (6)=i16 4 ("width (-)")) -> (F-format string=w348:string)  [unwired: 2 in]
            n78 = call "Oxford visa write read byte sized-- Hg.vi"("error in (no error)"=w339, "write buffer"="C3" ("Command"), "VISA resource name"=w338) -> ("error out"=w347:errorcluster, "VISA resource name out"=w344:refnum<visa-resource-name>)  [unwired: 6 in, 1 out]
            n79 = Concatenate Strings("D" ("string"), w348) -> (w350:string)
            n80 = call "Oxford visa write read byte sized-- Hg.vi"("error in (no error)"=w347, "write buffer"=w350, "VISA resource name"=w344) -> ("error out"=w340:errorcluster, "VISA resource name out"=w343:refnum<visa-resource-name>)  [unwired: 6 in, 1 out]
            n81 = call "Oxford visa write read byte sized-- Hg.vi"("error in (no error)"=w340, "write buffer"="C2" ("Command"), "VISA resource name"=w343) -> ("error out"=w341:errorcluster, "VISA resource name out"=w342:refnum<visa-resource-name>)  [unwired: 6 in, 1 out]
          }
        }
      }
      frame "heater auto" {
        n82 = case shown="\"enabled\"" w352 {
          tunnel: w359 -> [_ _]
          tunnel: w358 -> [w361 w365]
          tunnel: w357 -> [w360 w362]
          tunnel: [w360 w363] -> w356
          tunnel: [w361 w364] -> w355
          frame "disabled", Default {
          }
          frame "enabled" {
            n83 = call "Oxford visa write read byte sized-- Hg.vi"("error in (no error)"=w362, "write buffer"="C3" ("Command"), "VISA resource name"=w365) -> ("error out"=w372:errorcluster, "VISA resource name out"=w370:refnum<visa-resource-name>)  [unwired: 6 in, 1 out]
            n84 = call "Oxford visa write read byte sized-- Hg.vi"("error in (no error)"=w372, "write buffer"="A1" ("Command"), "VISA resource name"=w370) -> ("error out"=w366:errorcluster, "VISA resource name out"=w367:refnum<visa-resource-name>)  [unwired: 6 in, 1 out]
            n85 = call "Oxford visa write read byte sized-- Hg.vi"("error in (no error)"=w366, "write buffer"="C2" ("Command"), "VISA resource name"=w367) -> ("error out"=w363:errorcluster, "VISA resource name out"=w364:refnum<visa-resource-name>)  [unwired: 6 in, 1 out]
          }
        }
      }
      frame "heater manual and zero" {
        n86 = case shown="\"disabled\", Default" w374 {
          tunnel: w381 -> [_ _]
          tunnel: w380 -> [w383 w387]
          tunnel: w379 -> [w382 w386]
          tunnel: [w382 w385] -> w378
          tunnel: [w383 w384] -> w377
          frame "disabled", Default {
          }
          frame "enabled" {
            n87 = call "Oxford visa write read byte sized-- Hg.vi"("error in (no error)"=w386, "write buffer"="C3" ("Command"), "VISA resource name"=w387) -> ("error out"=w389:errorcluster, "VISA resource name out"=w392:refnum<visa-resource-name>)  [unwired: 6 in, 1 out]
            n88 = call "Oxford visa write read byte sized-- Hg.vi"("error in (no error)"=w389, "write buffer"="A0" ("Command"), "VISA resource name"=w392) -> ("error out"=w388:errorcluster, "VISA resource name out"=w391:refnum<visa-resource-name>)  [unwired: 6 in, 1 out]
            n89 = call "Oxford visa write read byte sized-- Hg.vi"("error in (no error)"=w388, "write buffer"="O000" ("Command"), "VISA resource name"=w391) -> ("error out"=w396:errorcluster, "VISA resource name out"=w395:refnum<visa-resource-name>)  [unwired: 6 in, 1 out]
            n90 = call "Oxford visa write read byte sized-- Hg.vi"("error in (no error)"=w396, "write buffer"="C2" ("Command"), "VISA resource name"=w395) -> ("error out"=w385:errorcluster, "VISA resource name out"=w384:refnum<visa-resource-name>)  [unwired: 6 in, 1 out]
          }
        }
      }
      frame "set heater to" {
        n91 = case shown="\"enabled\"" w399 {
          tunnel: w406 -> [_ w409]
          tunnel: w405 -> [w408 w417]
          tunnel: w404 -> [w407 w416]
          tunnel: [w407 w415] -> w403
          tunnel: [w408 w414] -> w402
          frame "disabled", Default {
          }
          frame "enabled" {
            (unwired) "O000" ("Command")
            n92 = Number To Fractional String(number=w409, precision (6)=i16 2) -> (F-format string=w411:string)  [unwired: 2 in]
            n93 = Concatenate Strings("O" ("Command"), w411) -> (w410:string)
            n94 = call "Oxford visa write read byte sized-- Hg.vi"("error in (no error)"=w416, "write buffer"="C3" ("Command"), "VISA resource name"=w417) -> ("error out"=w419:errorcluster, "VISA resource name out"=w422:refnum<visa-resource-name>)  [unwired: 6 in, 1 out]
            n95 = call "Oxford visa write read byte sized-- Hg.vi"("error in (no error)"=w419, "write buffer"="A0" ("Command"), "VISA resource name"=w422) -> ("error out"=w418:errorcluster, "VISA resource name out"=w421:refnum<visa-resource-name>)  [unwired: 6 in, 1 out]
            n96 = call "Oxford visa write read byte sized-- Hg.vi"("error in (no error)"=w418, "write buffer"=w410, "VISA resource name"=w421) -> ("error out"=w425:errorcluster, "VISA resource name out"=w424:refnum<visa-resource-name>)  [unwired: 6 in, 1 out]
            n97 = call "Oxford visa write read byte sized-- Hg.vi"("error in (no error)"=w425, "write buffer"="C2" ("Command"), "VISA resource name"=w424) -> ("error out"=w415:errorcluster, "VISA resource name out"=w414:refnum<visa-resource-name>)  [unwired: 6 in, 1 out]
          }
        }
      }
      frame "shut off" {
        n98 = case shown="\"enabled\"" w428 {
          tunnel: w435 -> [_ _]
          tunnel: w434 -> [w437 w447]
          tunnel: w433 -> [w436 w446]
          tunnel: [w436 w445] -> w432
          tunnel: [w437 w444] -> w431
          frame "disabled", Default {
          }
          frame "enabled" {
            w443 = 1.0  # Gas %
            # "stop sweep"
            # "Heater V = 0"
            # "Heater Manual"
            # "Remote"
            n99 = for {
              tunnel: string[] ["C3", "A0", "S0", "O000"] -> [w474] mode=indexing
              shift-right: [w472] -> w442
              shift-left: w447 -> [w475]
              shift-right: [w471] -> w441
              shift-left: w446 -> [w473]
              n100 = call "Oxford visa write read byte sized-- Hg.vi"("error in (no error)"=w473, "write buffer"=w474, "VISA resource name"=w475) -> ("error out"=w471:errorcluster, "VISA resource name out"=w472:refnum<visa-resource-name>)  [unwired: 6 in, 1 out]
            }
            n101 = case shown="True" TRUE {
              tunnel: w441 -> [w450 w457]
              tunnel: [w450 w456] -> w439
              tunnel: [w449 w453] -> w440
              tunnel: w442 -> [w449 w452]
              tunnel: w443 -> [_ w451]
              frame False {
                # "need to rize some kind of error ..."
              }
              frame True {
                n102 = call "Oxford visa write read byte sized-- Hg.vi"("error in (no error)"=w457, "write buffer"="C3" ("Command"), "VISA resource name"=w452) -> ("error out"=w461:errorcluster, "VISA resource name out"=w455:refnum<visa-resource-name>)  [unwired: 6 in, 1 out]
                n103 = Number To Fractional String(number=w451, precision (6)=i16 2) -> (F-format string=w462:string)  [unwired: 2 in]
                n104 = Concatenate Strings("G" ("string"), w462) -> (w459:string)
                n105 = call "Oxford visa write read byte sized-- Hg.vi"("error in (no error)"=w461, "write buffer"=w459, "VISA resource name"=w455) -> ("error out"=w460:errorcluster, "VISA resource name out"=w454:refnum<visa-resource-name>)  [unwired: 6 in, 1 out]
                n106 = call "Oxford visa write read byte sized-- Hg.vi"("error in (no error)"=w460, "write buffer"="C2" ("Command"), "VISA resource name"=w454) -> ("error out"=w456:errorcluster, "VISA resource name out"=w453:refnum<visa-resource-name>)  [unwired: 6 in, 1 out]
              }
            }
            n107 = disable-structure shown="Disabled" {
              disable-tunnel: w440 -> [w469 _]
              disable-tunnel: w439 -> [w468 _]
              disable-tunnel: [w467 _] -> w444
              disable-tunnel: [w466 _] -> w445
              frame Disabled {
                w470 = "C0"  # write buffer
                # "Local locked"
                n108 = call "Oxford visa write read byte sized-- Hg.vi"("error in (no error)"=w468, "write buffer"=w470, "VISA resource name"=w469) -> ("error out"=w466:errorcluster, "VISA resource name out"=w467:refnum<visa-resource-name>)  [unwired: 6 in, 1 out]
              }
              frame Enabled {
              }
            }
          }
        }
      }
      frame "test" {
      }
      frame "write sweep table" {
        n109 = case shown="\"enabled\"" w484 {
          tunnel: w491 -> [_ w494]
          tunnel: w490 -> [w493 w499]
          tunnel: w489 -> [w492 w498]
          tunnel: [w492 w496] -> w488
          tunnel: [w493 w495] -> w487
          tunnel: w483 -> [_ w497]
          frame "disabled", Default {
          }
          frame "enabled" {
            n110 = call "ITC 503 -- upload sweep table.vi"("error in"=w498, "Start set point"=w494, "Sweep Table"=w497, "ITC503 Address"=w499) -> ("error out"=w496:errorcluster, "ITC503 Address OUT"=w495:refnum<visa-resource-name>)  [unwired: 6 in]
          }
        }
      }
      frame "read state" {
        n111 = case shown="\"enabled\"" w503 {
          tunnel: [w509 w518] -> w508
          tunnel: w507 -> [w511 w517]
          tunnel: w506 -> [w510 w516]
          tunnel: [w510 w515] -> w505
          tunnel: [w511 w513] -> w504
          tunnel: w502 -> [w509 _]
          frame "disabled", Default {
          }
          frame "enabled" {
            w512 = u32 11 ("milliseconds -- wait time")
            w534 = FALSE
            n112 = case shown="True" w534 {
              tunnel: [w563 w568] -> w532
              tunnel: [w562 w567] -> w533
              tunnel: w517 -> [w563 w566]
              tunnel: w516 -> [w562 w565]
              tunnel: w512 -> [_ w564]
              frame False {
              }
              frame True {
                n113 = call "Oxford visa write read byte sized-- Hg.vi"("milliseconds -- wait time"=w564, "error in (no error)"=w565, "write buffer"="C3" ("Command"), "VISA resource name"=w566) -> ("error out"=w567:errorcluster, "VISA resource name out"=w568:refnum<visa-resource-name>)  [unwired: 5 in, 1 out]
              }
            }
            n114 = call "Oxford visa write read byte sized-- Hg.vi"("milliseconds -- wait time"=w512, "error in (no error)"=w533, "write buffer"="X", "VISA resource name"=w532) -> ("error out"=w528:errorcluster, "read buffer"=w519:string, "VISA resource name out"=w529:refnum<visa-resource-name>)  [unwired: 5 in]
            n115 = call "Oxford Read Channel -- Hg.vi"("milliseconds -- wait time"=w512, "error in (no error)"=w528, "Channel #"=1 ("Sensor #"), "VISA resource name"=w529) -> ("error out"=w535:errorcluster, "Data"=w525:dbl, "VISA resource name out"=w541:refnum<visa-resource-name>)  [unwired: 4 in, 1 out]
            n116 = call "Oxford Read Channel -- Hg.vi"("milliseconds -- wait time"=w512, "error in (no error)"=w535, "Channel #"=0 ("Sensor #"), "VISA resource name"=w541) -> ("error out"=w536:errorcluster, "Data"=w524:dbl, "VISA resource name out"=w542:refnum<visa-resource-name>)  [unwired: 4 in, 1 out]
            n117 = call "Oxford Read Channel -- Hg.vi"("milliseconds -- wait time"=w512, "error in (no error)"=w536, "Channel #"=6 ("Sensor #"), "VISA resource name"=w542) -> ("error out"=w537:errorcluster, "Data"=w523:dbl, "VISA resource name out"=w543:refnum<visa-resource-name>)  [unwired: 4 in, 1 out]
            n118 = call "Oxford Read Channel -- Hg.vi"("milliseconds -- wait time"=w512, "error in (no error)"=w537, "Channel #"=7 ("Sensor #"), "VISA resource name"=w543) -> ("error out"=w538:errorcluster, "Data"=w522:dbl, "VISA resource name out"=w544:refnum<visa-resource-name>)  [unwired: 4 in, 1 out]
            n119 = call "Oxford Read Channel -- Hg.vi"("milliseconds -- wait time"=w512, "error in (no error)"=w538, "Channel #"=8 ("Sensor #"), "VISA resource name"=w544) -> ("error out"=w539:errorcluster, "Data"=w521:dbl, "VISA resource name out"=w545:refnum<visa-resource-name>)  [unwired: 4 in, 1 out]
            n120 = call "Oxford Read Channel -- Hg.vi"("milliseconds -- wait time"=w512, "error in (no error)"=w539, "Channel #"=9 ("Sensor #"), "VISA resource name"=w545) -> ("error out"=w540:errorcluster, "Data"=w520:dbl, "VISA resource name out"=w546:refnum<visa-resource-name>)  [unwired: 4 in, 1 out]
            n121 = call "Oxford Read Channel -- Hg.vi"("milliseconds -- wait time"=w512, "error in (no error)"=w540, "Channel #"=10 ("Sensor #"), "VISA resource name"=w546) -> ("error out"=w531:errorcluster, "Data"=w514:dbl, "VISA resource name out"=w530:refnum<visa-resource-name>)  [unwired: 4 in, 1 out]
            n122 = case shown="True" w534 {
              tunnel: w530 -> [w554 w560]
              tunnel: w531 -> [w555 w559]
              tunnel: [w555 w558] -> w515
              tunnel: [w554 w557] -> w513
              tunnel: w512 -> [_ w556]
              frame False {
              }
              frame True {
                n123 = call "Oxford visa write read byte sized-- Hg.vi"("milliseconds -- wait time"=w556, "error in (no error)"=w559, "write buffer"="C2" ("Command"), "VISA resource name"=w560) -> ("error out"=w558:errorcluster, "VISA resource name out"=w557:refnum<visa-resource-name>)  [unwired: 5 in, 1 out]
              }
            }
            n124 = Bundle By Name(cluster=T1 {"ITC503 Address"="GPIB0::15::INSTR", "ITC temperature"=0.0, "ITC set temperature"=0.0, "heater"=0.0, "gas flow"=0.0, "P"=0.0, "D"=0.0, "I"=0.0, "ITC state"="", "nonzero temperature"=0.0, "Magn Field (T)"=0.0} ("itc box state OUT"), "ITC503 Address"=w513, "ITC temperature"=w525, "ITC set temperature"=w524, "heater"=w523, "gas flow"=w522, "P"=w521, "D"=w514, "I"=w520, "ITC state"=w519) -> (w518:T1)
          }
        }
      }
      frame "disable" {
      }
      frame "enable" {
      }
    }
  }
  "itc box state OUT" <- w6
  "Sweep Table" <- w10
  "enabled state" <- w7
  n125 = call <vilib>:"Check if File or Folder Exists.vi"("path"=w2) -> ("file or folder exists?"=w1:bool)  [unwired: 8 in, 2 out]
  n126 = case shown="True" w1 {
    tunnel: w4 -> [w582 w584]
    tunnel: [w582 w583] -> w3
    frame False {
    }
    frame True {
      w585 = TRUE  # Bypass Errors
      n127 = call "BypassAndLogErrors -- V2.vi"("Bypass Errors"=w585, "error in (no error)"=w584) -> ("error out"=w583:errorcluster)  [unwired: 9 in]
    }
  }
  "error out" <- w3
